vi "Compare Non-profile values.vi"(8 "error in (no error)":errorcluster, 11 "Non-profile parameter values":T1) -> (0 "error out":errorcluster)   [LabVIEW 2020]
uses:
  User Interface/User profiles code/Typedefs/Non-profile parameters cluster.ctl
  User Interface/User profiles code/Globals/gl_UsrProfiles globals.vi
panel:
  out "Parameter":string[](array[string])
  out "Changed":bool[](array[boolean])
  out "Current values":T1
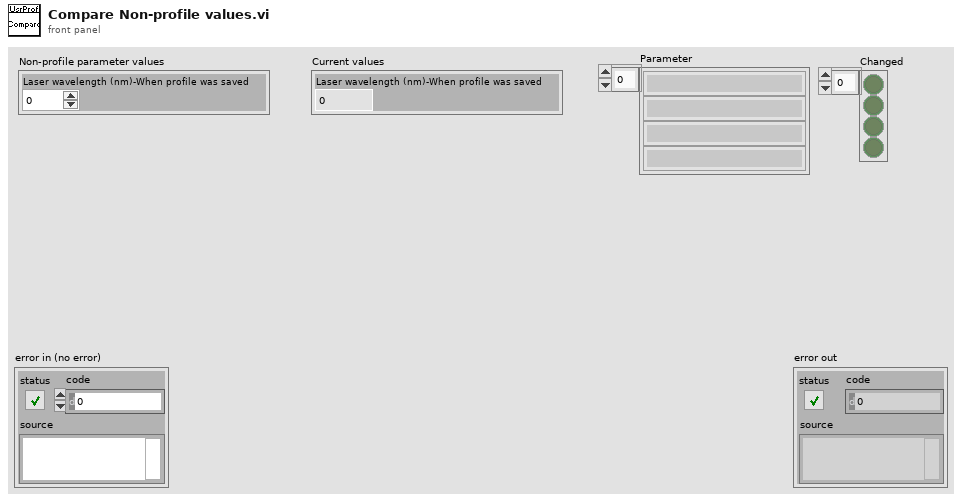
[diagram p1: front panel]
types:
  T1 = typedef "Non-profile parameters cluster.ctl" = cluster{"Laser wavelength (nm)-When profile was saved":dbl}
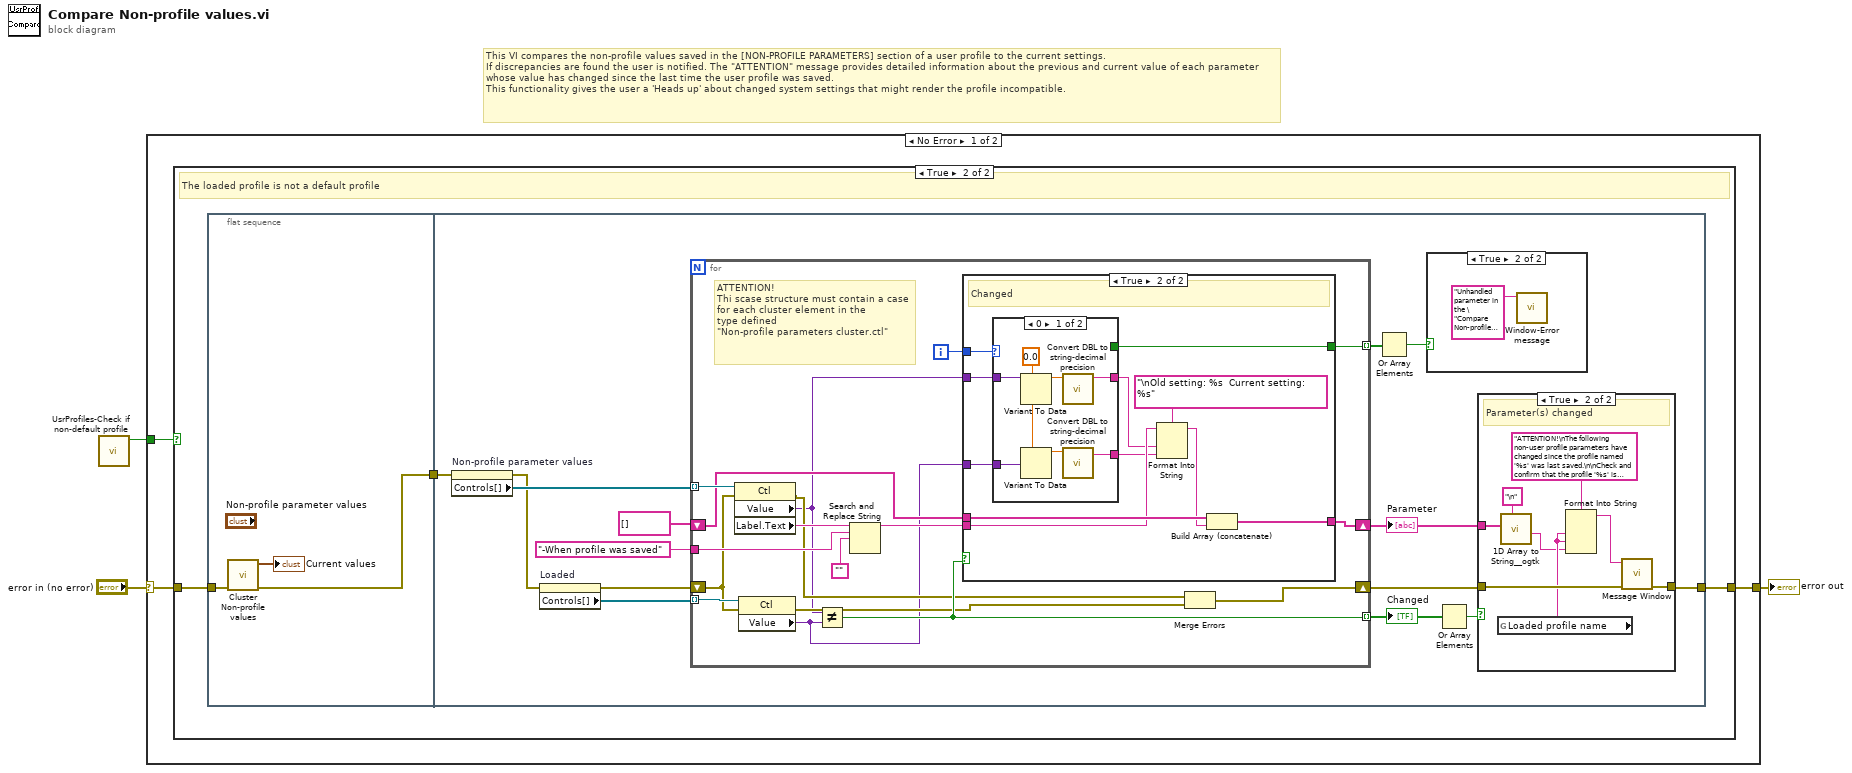
[diagram p0: block diagram]
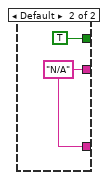
[diagram p6: hidden frame]
diagram:
  # "This VI compares the non-profile values saved in the [NON-PROFILE PARAMETERS] section of a user profile to the current settings.\nIf discrepancies are found the user is notified. The \"ATTENTION\" message provides detailed information about the previous and current value of each parameter whose value has changed since the last time the user profile was saved.\nThis functionality gives the user a 'Heads up' about changed system settings that might render the profile incompatible."
  n1 = call "UsrProfiles-Check if non-default profile.vi"() -> ("Non-default profile?"=w1:bool)  [unwired: 11 in]
  n2 = case shown="No Error" "error in (no error)" {
    selector: "error in (no error)" -> [w4 w76]
    tunnel: [w6 w76] -> w2
    tunnel: w1 -> [w5 _]
    frame No Error {
      n3 = case shown="True" w5 {
        tunnel: [w7 w9] -> w6
        tunnel: w4 -> [w7 w8]
        frame False {
          # "The loaded profile is a default profile"
        }
        frame True {
          # "The loaded profile is not a default profile"
          n4 = flat-sequence {
            tunnel: [w12] -> w10
            tunnel: w8 -> [w11]
            tunnel: w10 -> [w20]
            tunnel: [w16] -> w9
            frame #0 {
              n5 = call "Cluster Non-profile values.vi"("error in (no error)"=w11) -> ("error out"=w12:errorcluster, "Non-profile parameters cluster"=→"Current values":T1)  [unwired: 9 in]
            }
            frame #1 {
              n6 = property on="Non-profile parameter values" class="Clust (strict)"(error in=w20) -> (error out=w19:errorcluster, "Controls[]"=w27:refnum<vi>[])  [unwired: 1 in, 1 out]
              n7 = property on="Loaded" class="Clust (strict)"(error in=w19) -> (error out=w18:errorcluster, "Controls[]"=w26:refnum<vi>[])  [unwired: 1 in, 1 out]
              n8 = for {
                tunnel: w27 -> [w54] mode=indexing
                tunnel: w26 -> [w53] mode=indexing
                tunnel: [w49] -> w23 mode=indexing
                tunnel: "-When profile was saved" -> [w51]
                shift-right: [w38] -> w24
                shift-left: string[] [] -> [w47]
                shift-right: [w44] -> w17
                shift-left: w18 -> [w43]
                tunnel: [w39] -> w15 mode=indexing
                i -> [w42]
                # "ATTENTION!\nThi scase structure must contain a case for each cluster element in the \ntype defined \n\"Non-profile parameters cluster.ctl\""
                n9 = property class="Ctl"(reference=w54, error in=w43) -> (error out=w45:errorcluster, "Value"=w41:variant, "Label.Text"=w52:string)  [unwired: 1 out]
                n10 = property class="Ctl"(reference=w53, error in=w43) -> (error out=w46:errorcluster, "Value"=w40:variant)  [unwired: 1 out]
                n11 = Not Equal?(x=w41, y=w40) -> (x != y?=w49:bool)
                n12 = Search and Replace String(input string=w52, search string=w51, replace string="") -> (result string=w48:string)  [unwired: 5 in, 3 out]
                n13 = case shown="True" w49 {
                  tunnel: w48 -> [_ w61]
                  tunnel: [w55 w66] -> w38
                  tunnel: w47 -> [w55 w65]
                  tunnel: w42 -> [_ w64]
                  tunnel: w41 -> [_ w63]
                  tunnel: w40 -> [_ w62]
                  tunnel: [_ w58] -> w39
                  frame False {
                    # "No change"
                  }
                  frame True {
                    # "Changed"
                    n14 = case shown="0" w64 {
                      tunnel: w63 -> [w73 _]
                      tunnel: w62 -> [w70 _]
                      tunnel: [w68 w75] -> w56
                      tunnel: [w67 w75] -> w57
                      tunnel: [_ TRUE] -> w58
                      frame 0 {
                        w69 = 0.0 ("Laser wavelength (nm)-When profile was saved")
                        n15 = Variant To Data(type=w69, Variant=w73) -> (data=w72:dbl)  [unwired: 1 in, 1 out]
                        n16 = Variant To Data(type=w69, Variant=w70) -> (data=w71:dbl)  [unwired: 1 in, 1 out]
                        n17 = call <userlib>:"Convert DBL to string-decimal precision.vi"("DBL Value"=w72) -> ("Converted to String"=w67:string)  [unwired: 10 in]
                        n18 = call <userlib>:"Convert DBL to string-decimal precision.vi"("DBL Value"=w71) -> ("Converted to String"=w68:string)  [unwired: 10 in]
                      }
                      frame Default {
                        w75 = "N/A" ("Converted to String")
                      }
                    }
                    n19 = Format Into String(format string="\nOld setting: %s  Current setting: %s", initial string=w61, w57, w56) -> (resulting string=w60:string)  [unwired: 1 in, 1 out]
                    n20 = Build Array (concatenate)(w65, w60) -> (w66:string[])
                  }
                }
                n21 = Merge Errors(w45, w46) -> (w44:errorcluster)
              }
              "Changed" <- w23
              "Parameter" <- w24
              n22 = Or Array Elements(Boolean array=w15) -> (logical OR=w14:bool)
              n23 = case shown="True" w14 {
                frame False {
                }
                frame True {
                  n24 = call "Window-Error message.vi"("Message"="Unhandled parameter in the \"Compare Non-profile values.vi\"") -> ()  [unwired: 10 in, 1 out]
                }
              }
              n25 = Or Array Elements(Boolean array=w23) -> (logical OR=w21:bool)
              n26 = case shown="True" w21 {
                tunnel: w24 -> [_ w37]
                tunnel: w17 -> [w29 w34]
                tunnel: [w29 w33] -> w16
                frame False {
                }
                frame True {
                  # "Parameter(s) changed"
                  n27 = global read "gl_UsrProfiles globals.vi" "Loaded profile name"() -> (w31:string)
                  n28 = call <userlib>:"1D Array to String__ogtk.vi"("delimiter (Tab)"="\n", "Array of Strings"=w37) -> ("delimited string"=w30:string)  [unwired: 9 in]
                  n29 = Format Into String(format string="ATTENTION!\nThe following non-user profile parameters have changed since the profile named '%s' was last saved.\n\nCheck and confirm that the profile '%s' is compatible with the current settings shown at the end of this message.\n\nRe-save this profile if you do not want this message to appear each time this profile is loaded.\n\nCHANGED PARAMETER VALUES\n%s\n", w31, w31, w30) -> (resulting string=w32:string)  [unwired: 2 in, 1 out]
                  n30 = call "Message Window.vi"("error in (no error)"=w34, "Message string"=w32) -> ("error out (no error)"=w33:errorcluster)  [unwired: 9 in]
                }
              }
            }
          }
        }
      }
    }
    frame Error {
    }
  }
  "error out" <- w2
